vi "Example Math 1.vi"() -> ()   [LabVIEW 2014]
uses:
  <vilib>/LabVIEW Universal Transcriptor/LabVIEW for Arduino Math Library/Arduino Math.lvlib
panel:
  out "Error Out":errorcluster
  in  "Error In":errorcluster
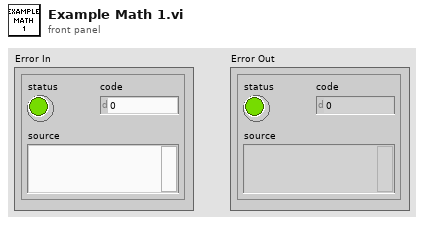
[diagram p1: front panel]
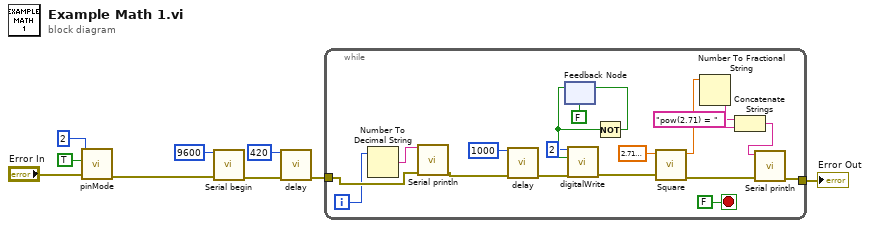
[diagram p0: block diagram]
diagram:
  n1 = call "pinMode.vi"("Error In"="Error In", "output?"=TRUE, "pin number"=2) -> ("Error Out"=w1:errorcluster)  [unwired: 8 in]
  n2 = call "Serial begin.vi"("Error In"=w1, "speed (Bd)"=9600) -> ("Error Out"=w8:errorcluster)  [unwired: 9 in]
  n3 = call "delay.vi"("Error In"=w8, "time (ms)"=420) -> ("Error Out"=w6:errorcluster)  [unwired: 9 in]
  n4 = while {
    tunnel: w6 -> [w26]
    tunnel: [w19] -> w5
    i -> [w18]
    stop <- FALSE stop-if-true
    n5 = Number To Decimal String(number=w18) -> (decimal integer string=w27:string)  [unwired: 1 in]
    n6 = call "Serial println.vi"("Error In"=w26, "string in"=w27) -> ("Error Out"=w24:errorcluster)  [unwired: 9 in]
    n7 = call "delay.vi"("Error In"=w24, "time (ms)"=1000) -> ("Error Out"=w23:errorcluster)  [unwired: 9 in]
    n8 = feedback #1(FALSE) -> (w21:bool)
    n9 = call "digitalWrite.vi"("Error In"=w23, "value"=w21, "pin number"=2) -> ("Error Out"=w16:errorcluster)  [unwired: 8 in]
    n10 = Not(x=w21) -> (.not. x?=w17:bool)
    n11 = feedback-in #1(w17) -> ()
    n12 = call <vilib>:"Square.vi"("Error In"=w16, "x"=sgl 2.71) -> ("Error Out"=w15:errorcluster, "x^2"=w13:sgl)  [unwired: 8 in]
    n13 = Number To Fractional String(number=w13) -> (F-format string=w11:string)  [unwired: 3 in]
    n14 = Concatenate Strings("pow(2.71) = " ("string"), w11) -> (w12:string)
    n15 = call "Serial println.vi"("Error In"=w15, "string in"=w12) -> ("Error Out"=w19:errorcluster)  [unwired: 9 in]
  }
  "Error Out" <- w5
